vi "Menu.BuildSubMenuTag.vi"(10 "Menu":string, 11 "Aliases Array":string[](array[string])) -> (3 "Tag Array":string[](array[string]))   [LabVIEW 2013, in "Simple Sequence Tools - Editor.lvlib"]
uses:
  Simple Sequence Tools - Editor.lvlib
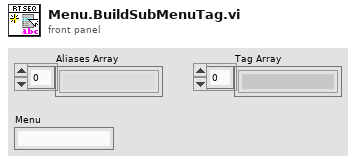
[diagram p1: front panel]
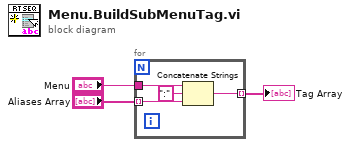
[diagram p0: block diagram]
diagram:
  n1 = for {
    tunnel: "Aliases Array" -> [w7] mode=indexing
    tunnel: "Menu" -> [w5]
    tunnel: [w4] -> w1 mode=indexing
    n2 = Concatenate Strings(w5, ":" ("string"), w7) -> (w4:string)
  }
  "Tag Array" <- w1
